vi "Run Test.vi"(8 "error in (no error)":errorcluster, 11 "Test Template in":refnum<class "Rocom LED Test.lvclass">) -> (0 "error out":errorcluster, 1 "Fail Codes":string[](array[string]), 2 "Tests Passed":bool[](array[boolean]), 3 "Test Template out":refnum<class "Rocom LED Test.lvclass">)   [LabVIEW 2015, in "Rocom LED Test.lvclass"]
uses:
  Rocom LED Test.lvclass
  Test Class/Test Class.lvclass
  Classes/Application/Class/Application.lvclass
  Classes/Manufacturing Test/Class/SC Manufacturing Test.lvclass
  Rocom Tests/Rocom Tests.lvclass
  <vilib>/Cree, Inc/Cree Test Framework/Classes/Base Objects/Base Class/Base Class/Base Class.lvclass
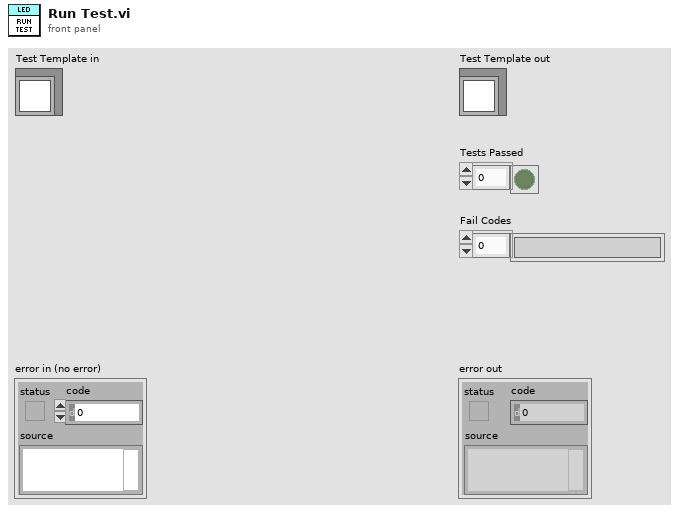
[diagram p1: front panel]
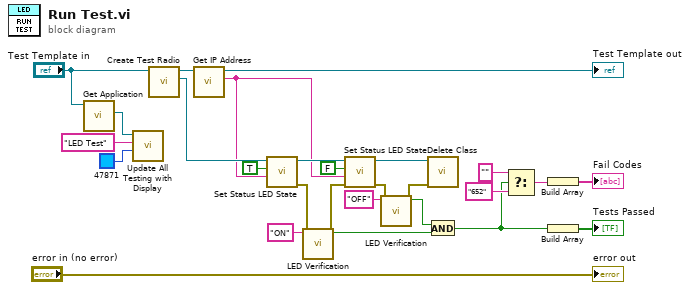
[diagram p0: block diagram]
diagram:
  n1 = call "Get Application.vi"("Test Class in"="Test Template in") -> ("Application.lvlib:Application.lvclass"=w27:refnum<class "Application.lvclass">)  [unwired: 9 in, 1 out]
  n2 = call "Update All Testing with Display.vi"("BG Color"=u32 47871, "Message ('')"="LED Test", "Application in"=w27) -> ()  [unwired: 7 in, 2 out]
  n3 = call "Create Test Radio.vi"("Rocom Tests in"="Test Template in") -> ("Test Radio"=w20:refnum<class "SC Manufacturing Test.lvclass">, "Rocom Tests out"=w19:refnum<class "Rocom LED Test.lvclass">)  [unwired: 8 in, 1 out]
  n4 = call "Get IP Address.vi"("Rocom Tests in"=w19) -> ("IP Address"=w18:string, "Rocom Tests out"=→"Test Template out":refnum<class "Rocom LED Test.lvclass">)  [unwired: 8 in, 1 out]
  n5 = call "Set Status LED State.vi"("IP Address"=w18, "State (Off)"=TRUE, "Acrobat Template in"=w20) -> ("error out"=w8:errorcluster, "Acrobat Template out"=w24:refnum<class "SC Manufacturing Test.lvclass">)  [unwired: 7 in]
  n6 = call "LED Verification.vi"("Error in"=w8, "String"="ON") -> ("Error out"=w7:errorcluster, "LED State"=w6:bool)  [unwired: 8 in]
  n7 = call "Set Status LED State.vi"("error in (no error)"=w7, "IP Address"=w18, "State (Off)"=FALSE, "Acrobat Template in"=w24) -> ("error out"=w5:errorcluster, "Acrobat Template out"=w17:refnum<class "SC Manufacturing Test.lvclass">)  [unwired: 6 in]
  n8 = call "LED Verification.vi"("Error in"=w5, "String"="OFF") -> ("Error out"=w4:errorcluster, "LED State"=w3:bool)  [unwired: 8 in]
  n9 = call <vilib>:"Delete Class.vi"("error in (no error)"=w4, "Base Class in"=w17) -> ()  [unwired: 8 in, 2 out]
  n10 = And(x=w3, y=w6) -> (x .and. y?=w13:bool)
  n11 = Select(t="", s=w13, f="652") -> (s? t:f=w11:string)
  n12 = Build Array(w11) -> (→"Fail Codes":string[])
  n13 = Build Array(w13) -> (→"Tests Passed":bool[])
  "error out" <- "error in (no error)"
